vi "Gaussmeter425_PositionScan.vi"() -> ()   [LabVIEW 2014]
uses:
  <instrlib>/Agilent 3446X Series/Public/Data/Read (Multiple Points).vi
  <instrlib>/Lake Shore 425/Public/Data/Field Data (Multiple Readings).vi
  <vilib>/Utility/file.llb/Write To Spreadsheet File (DBL).vi
  <instrlib>/Lake Shore 425/Lake Shore 425.lvlib
  <instrlib>/Agilent 3446X Series/Agilent 3446X Series.lvlib
  <vilib>/Analysis/NI_AALBase.lvlib
panel:
  out "?":cluster{dbl[], dbl[]}(graph)
  out "Current":cluster{dbl[], dbl[]}(graph)
  out "Measurement progress":u8(slide) scale=0.0..100.0
  out "Sigma I [A]":dbl
  out "Mean I  [A]":dbl
  in  "Readings per position":i32=5
  out "Position [mm]":dbl
  in  "Input file with positions":path
  in  "Reading Interval [ms]":i32=100
  in  "Readings per position":i32=10
  out "Sigma B [mT]":dbl
  out "Mean B [mT]":dbl
  out "Output file":string
  in  "Switch ON / OFF":bool=TRUE
  in  "VISA resource name MM":refnum<visa-resource-name>="USB0::0x0957::0x1A07::MY53203201::INSTR"
  in  "Measurement Function (10: Voltage DC)":i32(ring)=10 items=["Continuity", "Current AC", "Current DC", "Diode", "Frequency", "Resistance 4-wire", "Period", "Resistance 2-wire", "Temperature", "Voltage AC", "Voltage DC", "Voltage DC Ratio"]
  in  "VISA resource name GM":refnum<visa-resource-name>="COM4"
  in  "Serial Configuration":T1={"Baud Rate"=57600, "Parity"=1, "Data Bits"=7, "Stop Bits"=10, "Flow Control"=0} {"Flow Control" items=["None", "XON/XOFF", "RTS/CTS", "XON/XOFF & RTS/CTS", "DTR/DSR", "XON/XOFF & DTR/DSR"]; "Stop Bits" items=["1.0"=10, "1.5"=15, "2.0"=20]; "Data Bits" items=["7"=7, "8"=8]; "Parity" items=["None", "Odd", "Even", "Mark", "Space"]; "Baud Rate" items=["300"=300, "600"=600, "1200"=1200, "2400"=2400, "4800"=4800, "9600"=9600, "19200"=19200, "38400"=38400, "57600"=57600]}
  # "Measurement at current position"
  # "Gaussmeter"
  # "Multimeter"
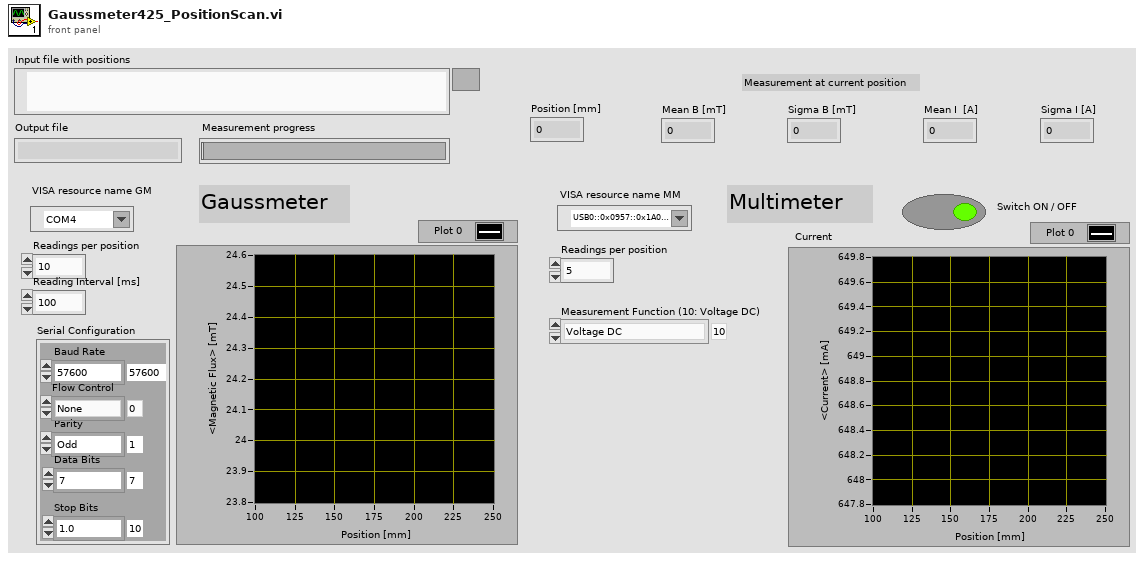
[diagram p1: front panel]
types:
  T1 = cluster{"Baud Rate":u32, "Parity":u16, "Data Bits":u16, "Stop Bits":u16, "Flow Control":u16}
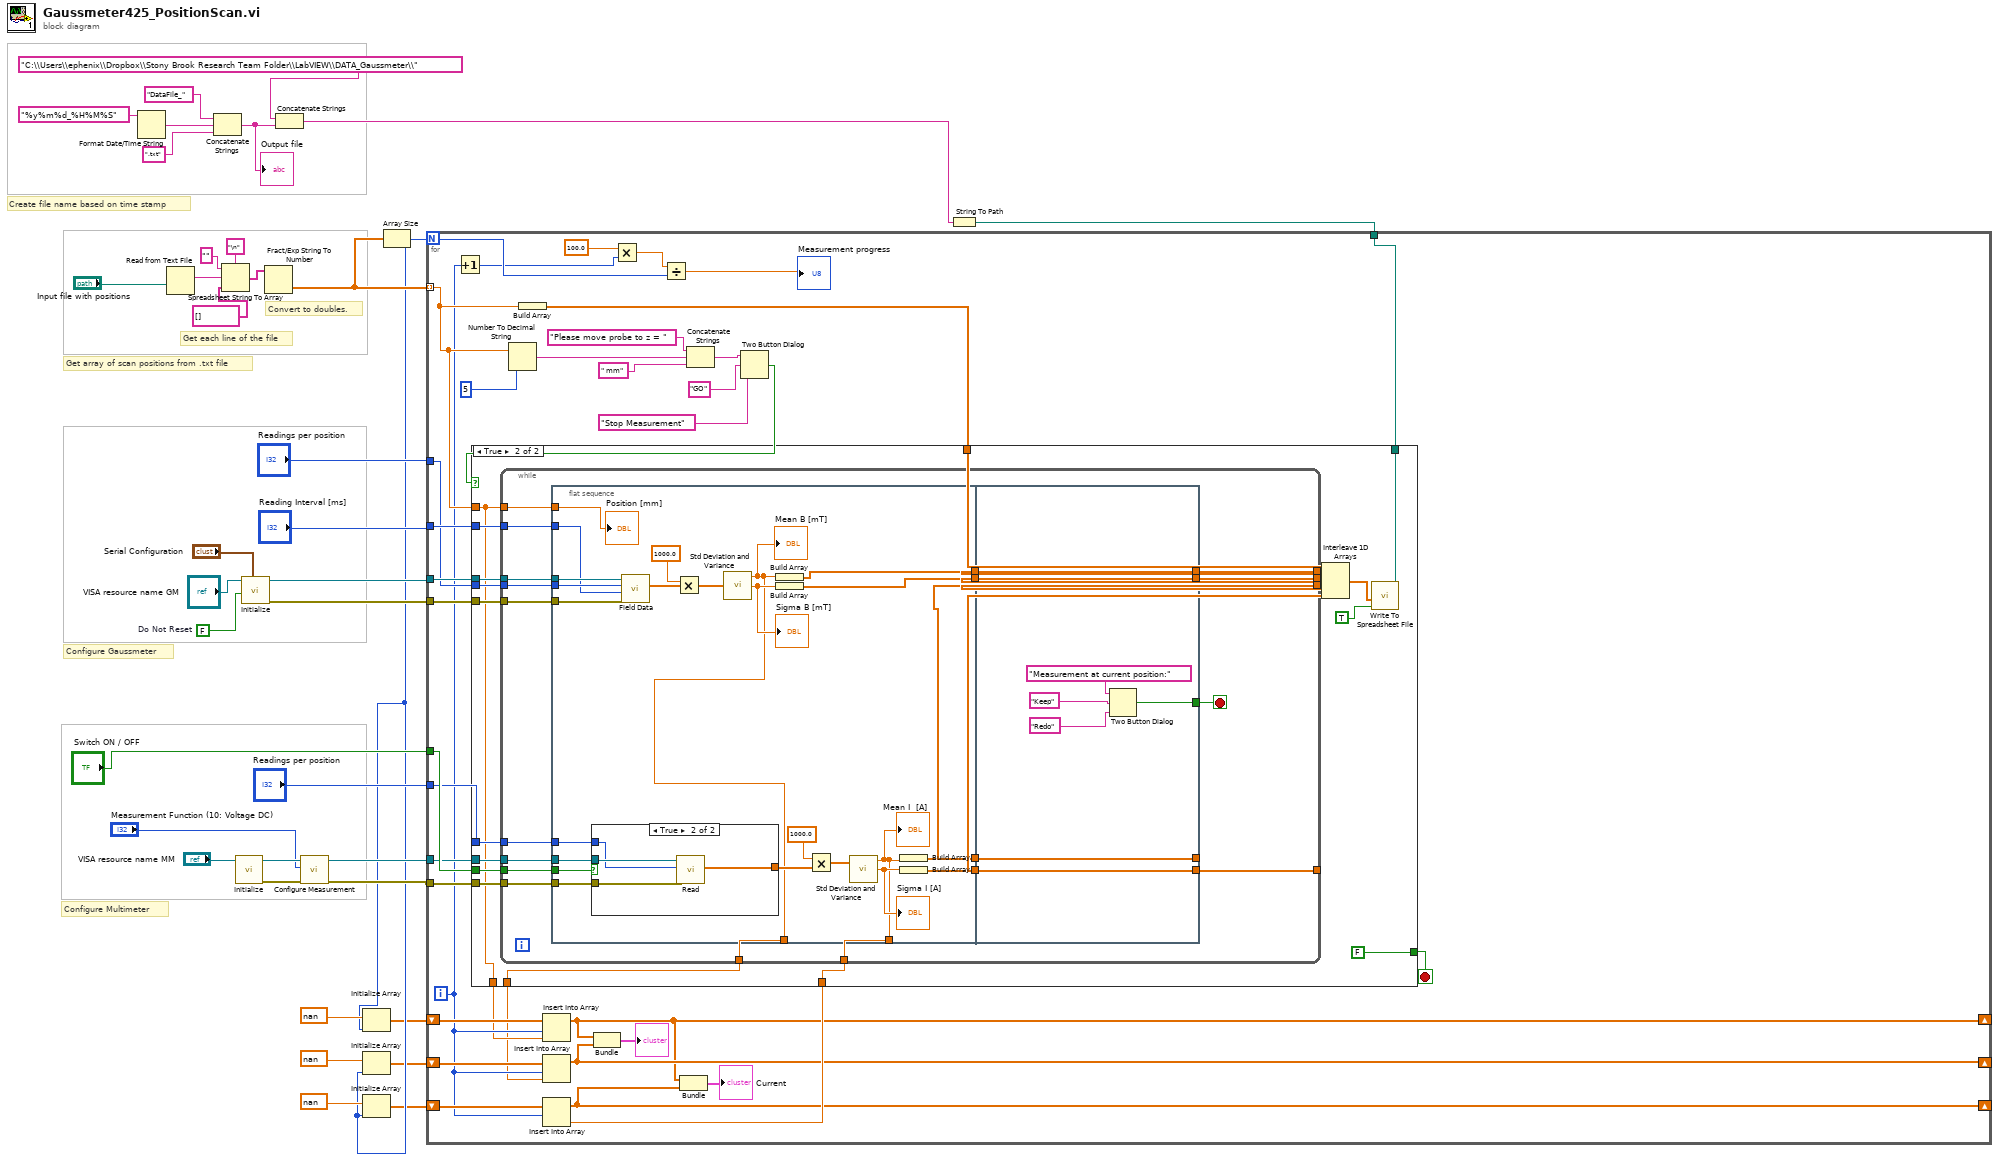
[diagram p0: block diagram]
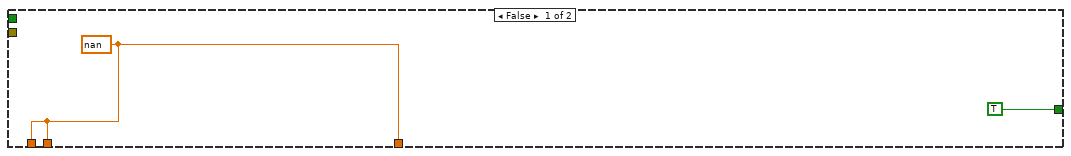
[diagram p2: hidden frame]
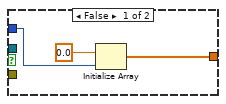
[diagram p3: hidden frame]
diagram:
  w36 = FALSE  # Do Not Reset
  # "Configure Multimeter"
  # "Configure Gaussmeter"
  # "Get array of scan positions from .txt file"
  # "Convert to doubles."
  # "Get each line of the file"
  # "Create file name based on time stamp"
  n1 = Format Date/Time String(time format string (%c)="%y%m%d_%H%M%S") -> (date/time string=w29:string)  [unwired: 2 in]
  n2 = Read from Text File(file (use dialog)="Input file with positions") -> (text=w16:string)  [unwired: 1 in, 5 out]
  n3 = Concatenate Strings("DataFile_", w29, ".txt") -> (w20:string)
  "Output file" <- w20
  n4 = Spreadsheet String To Array(delimiter (Tab)="\n", format string="", spreadsheet string=w16, array type (2D Dbl)=string[] []) -> (array=w10:string[])
  n5 = call <instrlib>:"Initialize.vi"("VISA resource name"="VISA resource name MM") -> ("error out"=w26:errorcluster, "VISA resource name out"=w27:refnum<visa-resource-name>)  [unwired: 4 in, 5 out]
  n6 = call <instrlib>:"Initialize.vi"("Serial Configuration"="Serial Configuration", "Reset (True)"=w36, "VISA resource name"="VISA resource name GM") -> ("error out"=w33:errorcluster, "VISA resource name out"=w34:refnum<visa-resource-name>)  [unwired: 7 in]
  n7 = Fract/Exp String To Number(string=w10) -> (number=w9:dbl[])  [unwired: 4 out]
  n8 = Concatenate Strings("C:\\Users\\ephenix\\Dropbox\\Stony Brook Research Team Folder\\LabVIEW\\DATA_Gaussmeter\\", w20) -> (w11:string)
  n9 = call <instrlib>:"Configure Measurement.vi"("error in (no error)"=w26, "Measurement Function (10: Voltage DC)"="Measurement Function (10: Voltage DC)", "VISA resource name"=w27) -> ("error out"=w22:errorcluster, "VISA resource name out"=w23:refnum<visa-resource-name>)  [unwired: 3 in, 4 out]
  n10 = Array Size(array=w9) -> (size(s)=w4:i32)
  n11 = Initialize Array(nan, w4) -> (w3:dbl[])
  n12 = Initialize Array(nan, w4) -> (w2:dbl[])
  n13 = Initialize Array(nan, w4) -> (w1:dbl[])
  n14 = String To Path(string=w11) -> (path=w12:path)
  n15 = for {
    N: w4 -> [w52]
    tunnel: w34 -> [w74]
    tunnel: w33 -> [w73]
    tunnel: w23 -> [w65]
    tunnel: w22 -> [w72]
    tunnel: "Switch ON / OFF" -> [w71]
    tunnel: "Reading Interval [ms]" -> [w70]
    tunnel: "Readings per position" -> [w69]
    tunnel: w12 -> [w67]
    tunnel: w9 -> [w60] mode=indexing
    tunnel: "Readings per position" -> [w68]
    shift-right: [w40] -> _
    shift-left: w3 -> [w50]
    shift-right: [w42] -> _
    shift-left: w2 -> [w48]
    shift-right: [w39] -> _
    shift-left: w1 -> [w49]
    i -> [w46]
    stop <- w56 stop-if-true
    n16 = Increment(x=w46) -> (x+1=w47:i32)
    n17 = Number To Decimal String(number=w60, width (-)=5) -> (decimal integer string=w62:string)
    n18 = Build Array(w60) -> (w66:dbl[])
    n19 = Multiply(x=100.0, y=w47) -> (x*y=w54:dbl)
    n20 = Divide(x=w54, y=w52) -> (x/y=→"Measurement progress":dbl)
    n21 = Concatenate Strings("Please move probe to z = ", w62, " mm") -> (w58:string)
    n22 = Two Button Dialog(message=w58, 1:"Stop Measurement", 2:"GO") -> (T button?=w59:bool)
    n23 = case shown="True" w59 {
      tunnel: w74 -> [_ w96]
      tunnel: w73 -> [_ w95]
      tunnel: w72 -> [_ w94]
      tunnel: w71 -> [_ w93]
      tunnel: w70 -> [_ w92]
      tunnel: w69 -> [_ w91]
      tunnel: w68 -> [_ w90]
      tunnel: w67 -> [_ w87]
      tunnel: w66 -> [_ w81]
      tunnel: w65 -> [_ w83]
      tunnel: w60 -> [_ w79]
      tunnel: [TRUE FALSE] -> w56
      tunnel: [w75 w79] -> w45
      tunnel: [w75 w78] -> w44
      tunnel: [w75 w77] -> w43
      frame False {
        w75 = nan
      }
      frame True {
        n24 = while {
          tunnel: w96 -> [w116]
          tunnel: w95 -> [w115]
          tunnel: w94 -> [w114]
          tunnel: w93 -> [w113]
          tunnel: w92 -> [w102]
          tunnel: w91 -> [w103]
          tunnel: w90 -> [w112]
          tunnel: [w111] -> w86
          tunnel: [w110] -> w85
          tunnel: [w109] -> w84
          tunnel: w83 -> [w108]
          tunnel: [w107] -> w80
          tunnel: w79 -> [w106]
          tunnel: [w105] -> w78
          tunnel: [w104] -> w77
          stop <- w97 stop-if-true
          n25 = flat-sequence {
            tunnel: w116 -> [w139]
            tunnel: w115 -> [w138]
            tunnel: w114 -> [w137]
            tunnel: w113 -> [w136]
            tunnel: w112 -> [w134]
            tunnel: w108 -> [w124]
            tunnel: w106 -> [w121]
            tunnel: [w120] -> w105
            tunnel: [w119] -> w104
            tunnel: w103 -> [w118]
            tunnel: w102 -> [w117]
            tunnel: [w131] -> w101
            tunnel: [w130] -> w100
            tunnel: [w129] -> w99
            tunnel: [w122] -> w98
            tunnel: [w151] -> w107
            tunnel: [w152] -> w109
            tunnel: [w153] -> w110
            tunnel: [w154] -> w111
            tunnel: w101 -> [w154]
            tunnel: w100 -> [w153]
            tunnel: w99 -> [w152]
            tunnel: w98 -> [w151]
            tunnel: [w147] -> w97
            frame #0 {
              n26 = case shown="True" w136 {
                tunnel: [w141 w146] -> w135
                tunnel: w137 -> [_ w145]
                tunnel: w124 -> [_ w144]
                tunnel: w134 -> [w140 w143]
                frame False {
                  n27 = Initialize Array(0.0, w140) -> (w141:dbl[])
                }
                frame True {
                  n28 = call-poly <instrlib>:"Read.vi"("error in (no error)"=w145, "Sample Count (1)"=w143, "VISA resource name"=w144) -> ("Measurements"=w146:dbl[])  [unwired: 1 in, 7 out]
                }
              }
              n29 = call-poly <instrlib>:"Field Data.vi"("error in (no error)"=w138, "Reading Interval (100)"=w117, "Sample Count (1)"=w118, "VISA resource name"=w139) -> ("Field Readings"=w128:dbl[])  [unwired: 5 in, 2 out]
              n30 = Multiply(x=1000.0, y=w128) -> (x*y=w127:dbl[])
              n31 = call <vilib>:"Std Deviation and Variance.vi"("X"=w127) -> ("mean"=w120:dbl, "standard deviation"=w132:dbl)  [unwired: 1 in, 1 out]
              "Mean B [mT]" <- w120
              "Sigma B [mT]" <- w132
              n32 = Build Array(w120) -> (w122:dbl[])
              n33 = Build Array(w132) -> (w131:dbl[])
              n34 = Multiply(x=1000.0, y=w135) -> (x*y=w133:dbl[])
              n35 = call <vilib>:"Std Deviation and Variance.vi"("X"=w133) -> ("mean"=w119:dbl, "standard deviation"=w123:dbl)  [unwired: 1 in, 1 out]
              "Mean I  [A]" <- w119
              "Sigma I [A]" <- w123
              n36 = Build Array(w119) -> (w130:dbl[])
              n37 = Build Array(w123) -> (w129:dbl[])
              "Position [mm]" <- w121
            }
            frame #1 {
              n38 = Two Button Dialog(message="Measurement at current position:", 1:"Redo", 2:"Keep") -> (T button?=w147:bool)
            }
          }
        }
        n39 = Interleave 1D Arrays(w81, w80, w86, w85, w84) -> (w89:dbl[])
        n40 = call-poly <vilib>:"Write To Spreadsheet File.vi"("append to file? (new file:F)"=TRUE, "1D data"=w89, "file path (dialog if empty)"=w87) -> ()  [unwired: 5 in, 1 out]
      }
    }
    n41 = Insert Into Array(array=w50, index=w46, new element=w45) -> (w40:dbl[])
    n42 = Insert Into Array(array=w48, index=w46, new element=w44) -> (w42:dbl[])
    n43 = Insert Into Array(array=w49, index=w46, new element=w43) -> (w39:dbl[])
    n44 = Bundle(w40, w42) -> (→"?":cluster{dbl[], dbl[]})  [unwired: 1 in]
    n45 = Bundle(w40, w39) -> (→"Current":cluster{dbl[], dbl[]})  [unwired: 1 in]
  }
